vi "Get all results as 1D strings array.vi"(8 "error in (no error)":errorcluster, 11 "PQ Result in":refnum<class "PQ Result.lvclass">) -> (0 "error out":errorcluster, 2 "Strings (Rows or Columns)":string[](array[string]), 3 "PQ Result out":refnum<class "PQ Result.lvclass">)   [LabVIEW 2013, in "PQ Result.lvclass"]
uses:
  PQ Result.lvclass
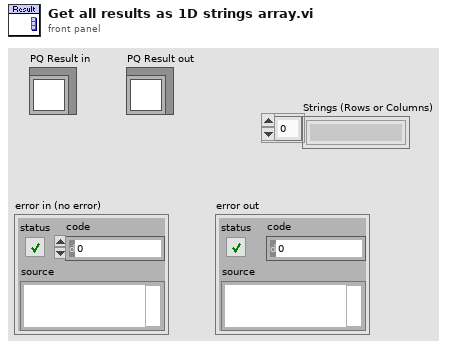
[diagram p1: front panel]
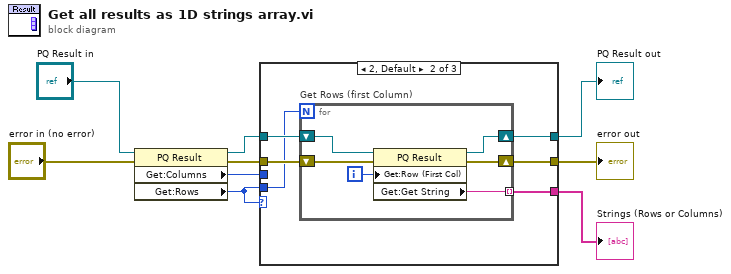
[diagram p0: block diagram]
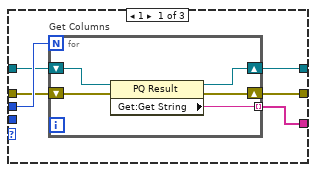
[diagram p2: hidden frame]
diagram:
  n1 = property class="PQ Result"(reference="PQ Result in", error in="error in (no error)") -> (reference out=w7:refnum<class "PQ Result.lvclass">, error out=w3:errorcluster, "Get:Columns"=w9:i32, "Get:Rows"=w1:i32)
  n2 = case shown="2, Default" w1 {
    tunnel: w9 -> [w15 _ _]
    tunnel: [w14 w26 w34] -> w8
    tunnel: w1 -> [_ w21 _]
    tunnel: w7 -> [w11 w23 w34]
    tunnel: [w13 w25 _] -> w6
    tunnel: w3 -> [w10 w22 w33]
    tunnel: [w12 w24 w33] -> w2
    frame 1 {
      n3 = for "Get Columns" {
        N: w15 -> [_]
        shift-right: [w19] -> w14
        shift-left: w11 -> [w20]
        tunnel: [w18] -> w13 mode=indexing
        shift-right: [w16] -> w12
        shift-left: w10 -> [w17]
        n4 = property class="PQ Result"(reference=w20, error in=w17) -> (reference out=w19:refnum<class "PQ Result.lvclass">, error out=w16:errorcluster, "Get:Get String"=w18:string)
      }
    }
    frame 2, Default {
      n5 = for "Get Rows (first Column)" {
        N: w21 -> [_]
        shift-right: [w31] -> w26
        shift-left: w23 -> [w32]
        tunnel: [w30] -> w25 mode=indexing
        shift-right: [w28] -> w24
        shift-left: w22 -> [w29]
        i -> [w27]
        n6 = property class="PQ Result"(reference=w32, error in=w29, "Get:Row (First Col)"=w27) -> (reference out=w31:refnum<class "PQ Result.lvclass">, error out=w28:errorcluster, "Get:Get String"=w30:string)
      }
    }
    frame ..0 {
    }
  }
  "PQ Result out" <- w8
  "Strings (Rows or Columns)" <- w6
  "error out" <- w2
